vi "Proceed Image.vi"(8 "error in (no error)":errorcluster, 10 "Image":T1, 11 "IMAQ Display in":refnum<class "HIJ Vision Display.lvclass">) -> (0 "error out":errorcluster, 3 "HIJ Vision Display out":refnum<class "HIJ Vision Display.lvclass">)   [LabVIEW 2014, in "HIJ Vision Display.lvlib" / "HIJ Vision Display.lvclass"]
doc: "Das VI wird bei jedem neuen Bild aufgerufen. \nEs ist eine Statische Aktion des Aktors. Damit soll sichergestellt sein,\ndass Pre Process.vi vor dem Analyze.vi aufgerufen wird. \n\nPre Process zeitg Standarausgeben wie Ziel- und Schwerpunktkreuz. \nAlte Overlays werden gelöscht. Die Kindklassen wie z.B. IMAQdx Display können Pre Process.vi\nerweitern und z.B. ein Hintergrundbild abziehen. Nach Preprocessing wird\ndas Bild angezeigt. Bis hierher ist die Operation synchron. Es wird davon ausgegangen, dass\nPreprocessing schnell genug ist, und vor dem nachkommenden Bild abgeschlossen wird.\n\nDas eigentliche Auswerten des Bildes wird in Analyze Actor (AA) ausgelagert. Analyze.vi schickt\neine asynchrone Nachricht an Analyze Actor. Wenn der AA fertig ist, schickt er eine Nachricht \nmit Ergebnissen zurück. Je nach Komplexität der Auswertung, kann es passieren, dass Display \nActor beriets ein neues Bild anzeigt. Diese Situation kann anhand der Bildnummernvergleiches\nerkannt werden."
uses:
  HIJ Vision Display.lvclass
  <vilib>/vision/Image Controls.llb/IMAQ Image.ctl
  HIJ Vision Display.lvclass/HIJ Vision Display.ctl
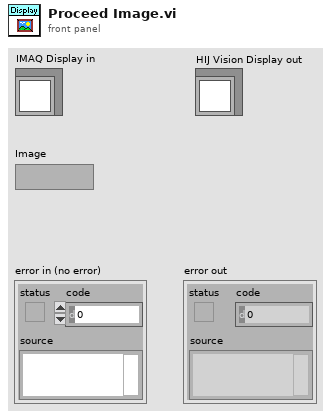
[diagram p1: front panel]
types:
  T1 = typedef "IMAQ Image.ctl" = refnum<image>
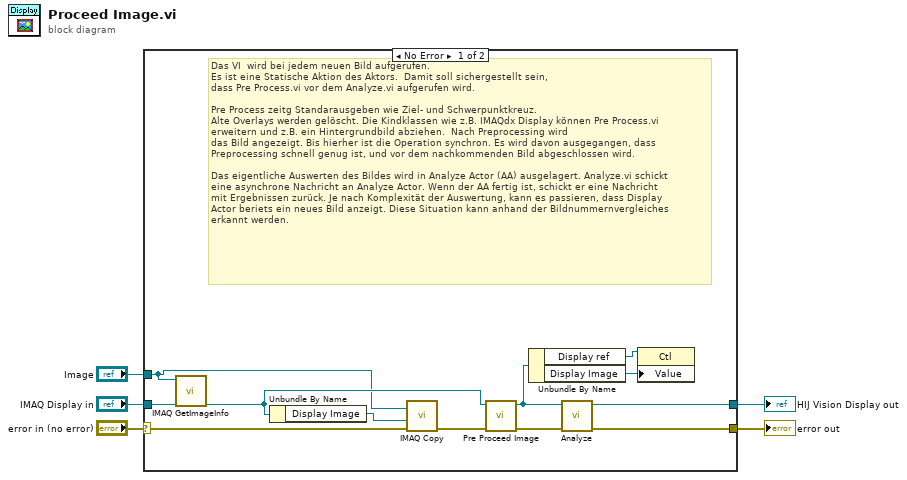
[diagram p0: block diagram]
diagram:
  n1 = case shown="No Error" "error in (no error)" {
    selector: "error in (no error)" -> [w14 w18]
    tunnel: [w15 w18] -> w4
    tunnel: "IMAQ Display in" -> [w16 w17]
    tunnel: "Image" -> [w6 _]
    tunnel: [w13 w17] -> w1
    frame No Error {
      # "Das VI  wird bei jedem neuen Bild aufgerufen. \nEs ist eine Statische Aktion des Aktors.  Damit soll sichergestellt sein,\ndass Pre Process.vi vor dem Analyze.vi aufgerufen wird. \n\nPre Process zeitg Standarausgeben wie Ziel- und Schwerpunktkreuz. \nAlte Overlays werden gelöscht. Die Kindklassen wie z.B. IMAQdx Display können Pre Process.vi\nerweitern und z.B. ein Hintergrundbild abziehen.  Nach Preprocessing wird\ndas Bild angezeigt. Bis hierher ist die Operation synchron. Es wird davon ausgegangen, dass\nPreprocessing schnell genug ist, und vor dem nachkommenden Bild abgeschlossen wird.\n\nDas eigentliche Auswerten des Bildes wird in Analyze Actor (AA) ausgelagert. Analyze.vi schickt\neine asynchrone Nachricht an Analyze Actor. Wenn der AA fertig ist, schickt er eine Nachricht \nmit Ergebnissen zurück. Je nach Komplexität der Auswertung, kann es passieren, dass Display \nActor beriets ein neues Bild anzeigt. Diese Situation kann anhand der Bildnummernvergleiches\nerkannt werden."
      n2 = call "IMAQ GetImageInfo"("Image"=w6) -> ()  [unwired: 3 in, 8 out]
      n3 = Unbundle By Name(w16) -> ("Display Image"=w7:T1)
      n4 = call "IMAQ Copy"("error in (no error)"=w14, "Image Dst"=w7, "Image Src"=w6) -> ("error out"=w10:errorcluster)  [unwired: 3 in, 1 out]
      n5 = call-dynamic "Pre Proceed Image.vi"("error in (no error)"=w10, "Display in"=w16) -> ("error out"=w9:errorcluster, "Display out"=w11:refnum<class "HIJ Vision Display.lvclass">)  [unwired: 8 in]
      n6 = Unbundle By Name(w11) -> ("Display ref"=w12:refnum<vi>, "Display Image"=w8:T1)
      n7 = call-dynamic "Analyze.vi"("error in (no error)"=w9, "HIJ Vision Display in"=w11) -> ("error out"=w15:errorcluster, "HIJ Vision Display out"=w13:refnum<class "HIJ Vision Display.lvclass">)  [unwired: 8 in]
      n8 = property class="Ctl"(reference=w12, "Value"=w8) -> ()  [unwired: 1 in, 2 out]
    }
    frame Error {
    }
  }
  "error out" <- w4
  "HIJ Vision Display out" <- w1
